vi "Build Feedback Message.vi"(8 "error in (no error)":errorcluster, 11 "Message":string) -> (0 "error out":errorcluster, 2 "Feedback":string, 3 "OK status":bool)   [LabVIEW 2021, in "Model_AMC.lvclass"]
uses:
  Model_AMC.lvclass
  Model_AMC.lvclass/Model_AMC.ctl
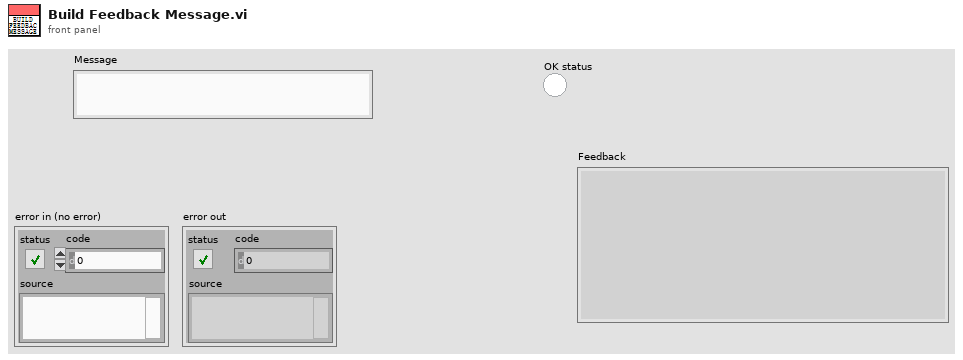
[diagram p1: front panel]
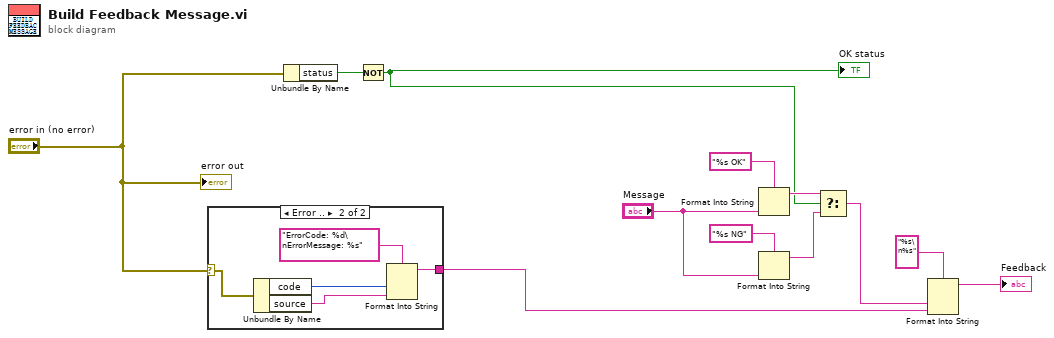
[diagram p0: block diagram]
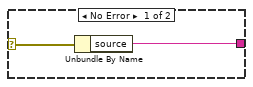
[diagram p2: hidden frame]
diagram:
  n1 = case shown="Error .." "error in (no error)" {
    selector: "error in (no error)" -> [w13 w15]
    tunnel: [w14 w16] -> w3
    frame No Error {
      n2 = Unbundle By Name(w13) -> ("source"=w14:string)
    }
    frame Error {
      n3 = Unbundle By Name(w15) -> ("code"=w18:i32, "source"=w19:string)
      n4 = Format Into String(format string="ErrorCode: %d\nErrorMessage: %s", w18, w19) -> (resulting string=w16:string)  [unwired: 2 in, 1 out]
    }
  }
  n5 = Unbundle By Name("error in (no error)") -> ("status"=w11:bool)
  n6 = Not(x=w11) -> (.not. x?=w6:bool)
  "OK status" <- w6
  n7 = Format Into String(format string="%s OK", "Message") -> (resulting string=w8:string)  [unwired: 2 in, 1 out]
  n8 = Format Into String(format string="%s NG", "Message") -> (resulting string=w10:string)  [unwired: 2 in, 1 out]
  n9 = Select(t=w8, s=w6, f=w10) -> (s? t:f=w2:string)
  n10 = Format Into String(format string="%s\n%s", w2, w3) -> (resulting string=→"Feedback":string)  [unwired: 2 in, 1 out]
  "error out" <- "error in (no error)"
